vi "CSM - Filter Interrupt Broadcasts.vi"(5 "States In":string) -> (6 "States Out":string)   [LabVIEW 2017, in "Communicable State Machine.lvlib"]
doc: "Filters interrupt broadcast messages in the CSM state queue.\n\n\n> [!NOTE] <b>CSM State Queue Operation API</b>\n>\n> This type of API only concatenates message strings and does not send messages directly. The message is sent and the operation executed within the Parse State Queue++ VI. Unlike the Message Building API, this type of API includes a CSM state queue string input, which is equivalent to inserting a message into the state queue.\n\n\n-- <b>Controls</b> --\n- <b>States In</b>: The entire state description string to filter.\n\n-- <b>Indicators</b> --\n- <b>States Out</b>: The filtered state description string."
uses:
  Communicable State Machine.lvlib
  _Shared/CSM Shared.lvlib
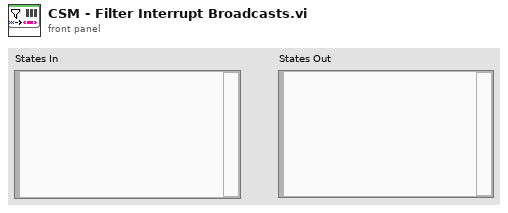
[diagram p1: front panel]
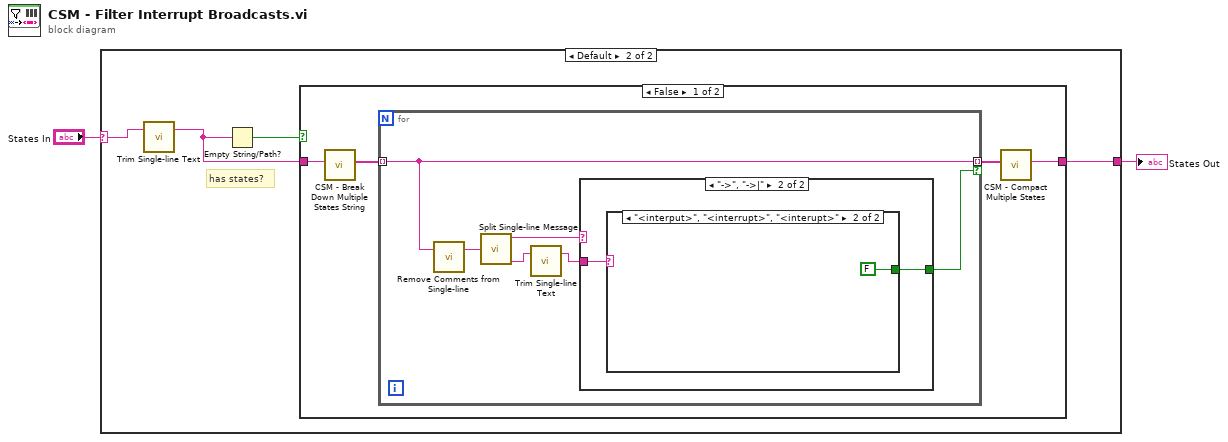
[diagram p0: block diagram]
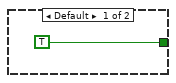
[diagram p3: hidden frame]
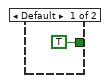
[diagram p4: hidden frame]
diagram:
  n1 = case shown="Default" "States In" {
    selector: "States In" -> [_ w3]
    tunnel: [_ w6] -> w1
    frame "" {
    }
    frame Default {
      # "has states?"
      n2 = call "Trim Single-line Text.vi"("single-line text"=w3) -> ("trimed text"=w4:string)  [unwired: 2 in]
      n3 = Empty String/Path?(string/path=w4) -> (empty?=w5:bool)
      n4 = case shown="False" w5 {
        tunnel: w4 -> [w10 w22]
        tunnel: [w9 w22] -> w6
        frame False {
          n5 = call "CSM - Break Down Multiple States String.vi"("States"=w10) -> ("Multiple States"=w8:string[])  [unwired: 10 in]
          n6 = for {
            tunnel: w8 -> [w15] mode=indexing
            tunnel: [w15] -> w7 mode=indexing if=w13
            n7 = call "Remove Comments from Single-line.vi"("single-line text"=w15) -> ("single-line text without comments"=w16:string)  [unwired: 2 in]
            n8 = call "Split Single-line Message.vi"("single-line text"=w16) -> ("operator"=w14:string, "source/target"=w12:string)  [unwired: 6 in, 2 out]
            n9 = call "Trim Single-line Text.vi"("single-line text"=w12) -> ("trimed text"=w11:string)  [unwired: 2 in]
            n10 = case shown="\"->\", \"->|\"" w14 {
              tunnel: [TRUE w19] -> w13
              tunnel: w11 -> [_ w18]
              frame Default {
              }
              frame "->", "->|" {
                n11 = case shown="\"<interput>\", \"<interrupt>\", \"<interupt>\"" w18 {
                  tunnel: [TRUE FALSE] -> w19
                  frame Default {
                  }
                  frame "<interput>", "<interrupt>", "<interupt>" {
                  }
                }
              }
            }
          }
          n12 = call "CSM - Compact Multiple States.vi"("Multiple States"=w7) -> ("States"=w9:string)  [unwired: 9 in]
        }
        frame True {
        }
      }
    }
  }
  "States Out" <- w1
